vi "pot_digit.vi"() -> ()   [LabVIEW 2014]
doc: "Digital pot: controlla il DS1804 con i DIO 0 -2\n0 = CB52 = CS\n1 = CB17 = U/D\n2 = CB49 =INC"
uses:
  <vilib>/DAQmx/write.llb/DAQmx Write (Digital 2D Bool NChan 1Samp NLine).vi
  <vilib>/DAQmx/write.llb/DAQmx Write (Digital Bool 1Line 1Point).vi
  <vilib>/DAQmx/create/channels.llb/DAQmx Create Channel (DO-Digital Output).vi
  <vilib>/DAQmx/miscellaneous.llb/DAQmx Fill In Error Info.vi
panel:
  in  "Numero inc":u32=10
  in  "data":bool[][](array[boolean])=[[TRUE, TRUE, FALSE]]
  # "CS"
  # "U/D"
  # "49      17     52"
  # "Utilizzare le linee  digitali 0,1,2 connesse a CS,  U/D  e INC :\n0 = CB 52 = CS\n1 = CB 17 = U/D\n2 = CB 49 = INC"
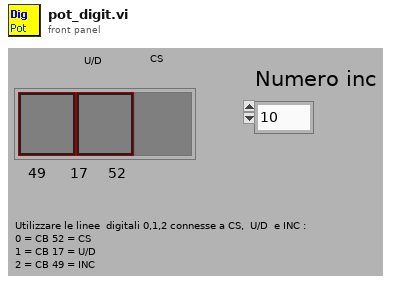
[diagram p1: front panel]
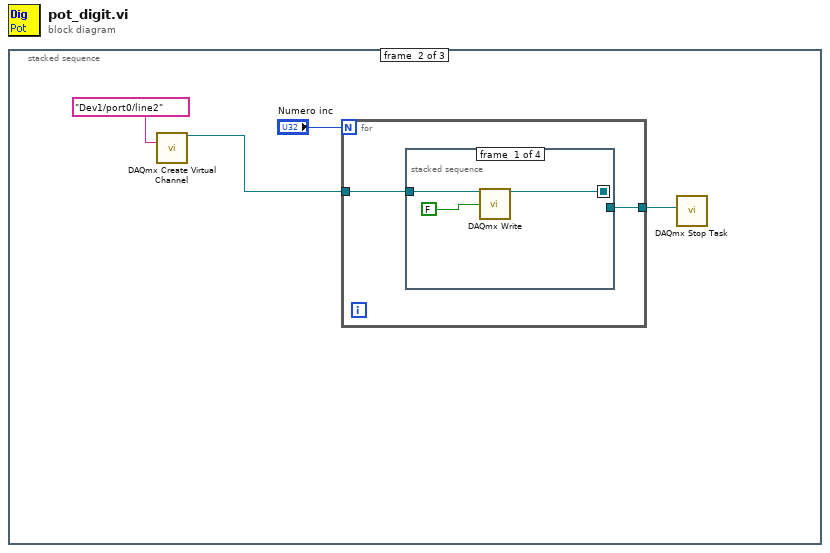
[diagram p0: block diagram]
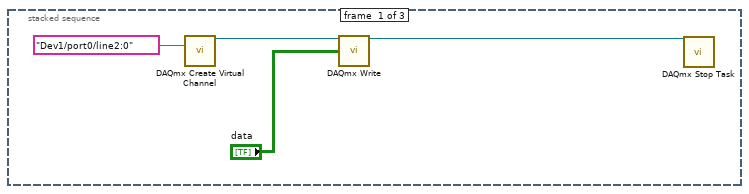
[diagram p2: hidden frame]
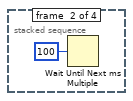
[diagram p3: hidden frame]
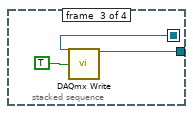
[diagram p4: hidden frame]
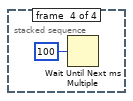
[diagram p5: hidden frame]
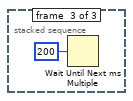
[diagram p6: hidden frame]
diagram:
  n1 = stacked-sequence {
    frame #0 {
      n2 = call-poly <vilib>:"DAQmx Create Virtual Channel.vi"("lines"=tag "Dev1/port0/line2:0" ("Scelta linee")) -> ("task out"=w3:refnum<k21>)  [unwired: 4 in, 10 out]
      n3 = call-poly <vilib>:"DAQmx Write.vi"("task/channels in"=w3, "data"="data") -> ("task out"=w1:refnum<k21>)  [unwired: 2 in, 11 out]
      n4 = call <vilib>:"DAQmx Stop Task.vi"("task/channels in"=w1) -> ()  [unwired: 1 in, 14 out]
    }
    frame #1 {
      n5 = call-poly <vilib>:"DAQmx Create Virtual Channel.vi"("lines"=tag "Dev1/port0/line2" ("Scelta linee  2")) -> ("task out"=w6:refnum<k21>)  [unwired: 4 in, 10 out]
      n6 = for {
        N: "Numero inc" -> [_]
        tunnel: w6 -> [w10]
        tunnel: [w9] -> w5
        n7 = stacked-sequence {
          seq-local: [w11 _ _ _] -> [_ _ w17 _]
          tunnel: w10 -> [w13 _ _ _]
          tunnel: [_ _ w15 _] -> w9
          frame #0 {
            n8 = call-poly <vilib>:"DAQmx Write.vi"("task/channels in"=w13, "data"=FALSE) -> ("task out"=w11:refnum<k21>)  [unwired: 2 in, 11 out]
          }
          frame #1 {
            n9 = Wait Until Next ms Multiple(millisecond multiple=u32 100) -> ()  [unwired: 1 out]
          }
          frame #2 {
            n10 = call-poly <vilib>:"DAQmx Write.vi"("task/channels in"=w17, "data"=TRUE) -> ("task out"=w15:refnum<k21>)  [unwired: 2 in, 11 out]
          }
          frame #3 {
            n11 = Wait Until Next ms Multiple(millisecond multiple=u32 100) -> ()  [unwired: 1 out]
          }
        }
      }
      n12 = call <vilib>:"DAQmx Stop Task.vi"("task/channels in"=w5) -> ()  [unwired: 1 in, 14 out]
    }
    frame #2 {
      n13 = Wait Until Next ms Multiple(millisecond multiple=u32 200) -> ()  [unwired: 1 out]
    }
  }
